vi "PAM Parse Sequence File.vi"(8 "error in":errorcluster, 11 "Sequence File":path) -> (0 "error out":errorcluster, 3 "Cluster Out":T1(array[cluster]))   [LabVIEW 2011]
uses:
  <vilib>/regexp/Match Regular Expression.xnode
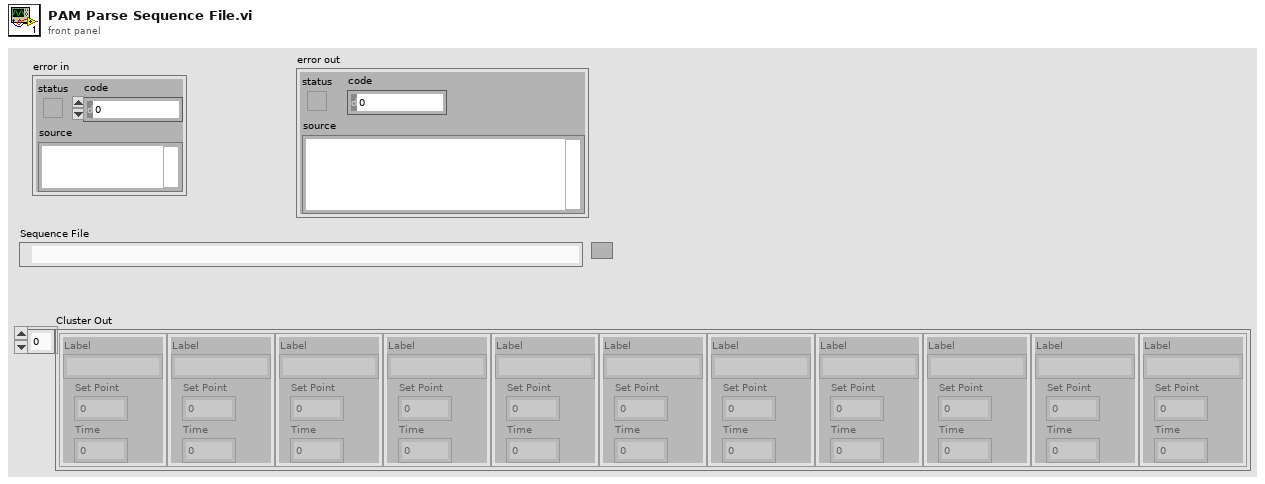
[diagram p1: front panel]
types:
  T1 = cluster{"Label":string, "Set Point":dbl, "Time":dbl}[]
  T2 = cluster{"Label":string, "Set Point":dbl, "Time":dbl}
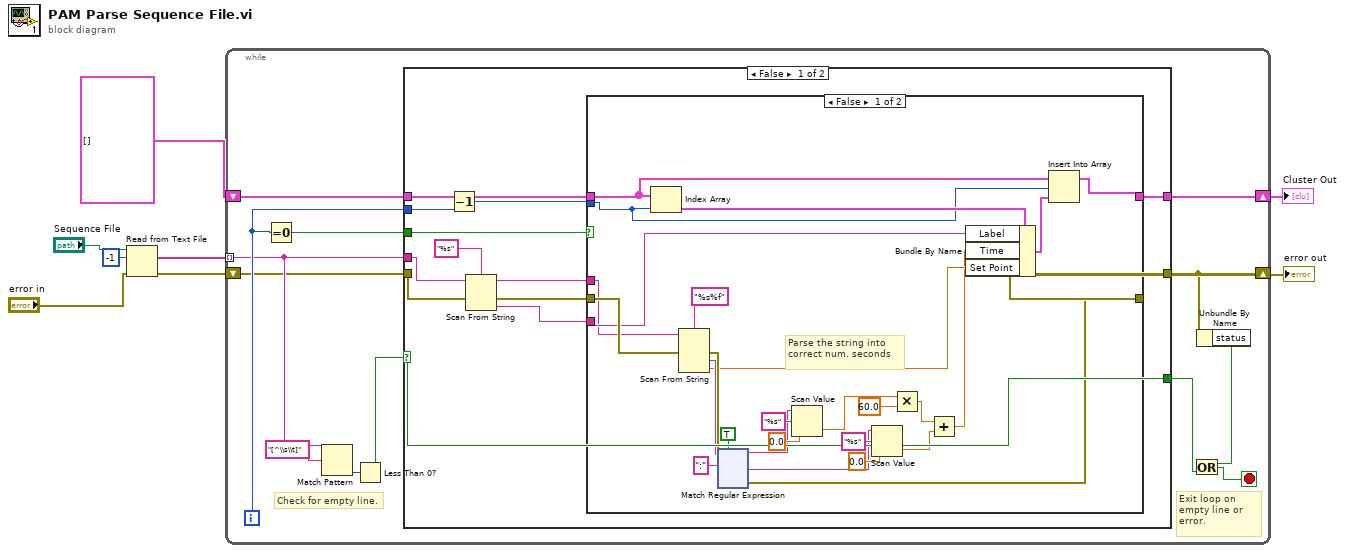
[diagram p0: block diagram]
diagram:
  n1 = Read from Text File(file (use dialog)="Sequence File", count=-1, error in="error in") -> (text=w6:string[], error out=w4:errorcluster)  [unwired: 1 in, 2 out]
  n2 = while {
    tunnel: w6 -> [w15] mode=indexing
    shift-right: [w13] -> w3
    shift-left: w4 -> [w14]
    shift-right: [w10] -> w1
    shift-left: T1 [] -> [w9]
    i -> [w17]
    stop <- w21 stop-if-true
    # "Exit loop on empty line or error."
    # "Check for empty line."
    n3 = Equal To 0?(x=w17) -> (x = 0?=w16:bool)
    n4 = Match Pattern(string=w15, regular expression="[^\\s\\t]") -> (offset past match=w19:i32)  [unwired: 1 in, 3 out]
    n5 = Less Than 0?(x=w19) -> (x < 0?=w18:bool)
    n6 = case shown="False" w18 {
      selector: w18 -> [w22 w175]
      tunnel: w17 -> [w34 _]
      tunnel: w16 -> [w32 _]
      tunnel: w15 -> [w31 _]
      tunnel: w14 -> [w30 w176]
      tunnel: [w23 w176] -> w13
      tunnel: [w22 w175] -> w11
      tunnel: [w25 w174] -> w10
      tunnel: w9 -> [w24 w174]
      frame False {
        n7 = Decrement(x=w34) -> (x-1=w33:i32)
        n8 = Scan From String(format string="%s", input string=w31, error in=w30) -> (remaining string=w28:string, error out=w29:errorcluster, output 1=w26:string)  [unwired: 2 in, 1 out]
        n9 = case shown="False" w32 {
          tunnel: w33 -> [w57 _]
          tunnel: w29 -> [w54 w173]
          tunnel: w28 -> [w52 _]
          tunnel: w26 -> [w53 _]
          tunnel: [w48 w173] -> w23
          tunnel: [w55 w172] -> w25
          tunnel: w24 -> [w56 w172]
          frame False {
            # "Parse the string into correct num. seconds"
            n10 = Index Array(array=w56, index=w57) -> (element=w59:T2)
            n11 = Scan From String(format string="%s%f", input string=w52, error in=w54) -> (error out=w49:errorcluster, output 1=w37:string, output 2=w36:dbl)  [unwired: 3 in, 2 out]
            n12 = xnode "Match Regular Expression"("input string"=w37, "regular expression"=":", "error in"=w49, "ignore case? (F)"=TRUE) -> ("before match"=w45:string, "after match"=w42:string, "error out"=w48:errorcluster)  [unwired: 2 in, 2 out]
            n13 = Scan Value(string=w45, format string="%s", default (0 dbl)=0.0) -> (value=w39:dbl)  [unwired: 1 out]
            n14 = Scan Value(string=w42, format string="%s", default (0 dbl)=0.0) -> (value=w38:dbl)  [unwired: 1 out]
            n15 = Multiply(x=w39, y=60.0) -> (x*y=w40:dbl)
            n16 = Add(x=w40, y=w38) -> (x+y=w35:dbl)
            n17 = Bundle By Name(cluster=w59, "Label"=w53, "Time"=w35, "Set Point"=w36) -> (w60:T2)
            n18 = Insert Into Array(array=w56, index=w57, new element=w60) -> (w55:T1)
          }
          frame True {
            # "Do nothing - this is the first line of the file, which is a comment."
          }
        }
      }
      frame True {
      }
    }
    n19 = Unbundle By Name(w13) -> ("status"=w12:bool)
    n20 = Or(x=w12, y=w11) -> (x .or. y?=w21:bool)
  }
  "error out" <- w3
  "Cluster Out" <- w1
